vi "niFpga wdp fft DIF 4spc.vi"(0 "real data in":fxp<+/-,8,1>[](array[numeric])=[0.0, 0.0, 0.0, 0.0], 5 "imaginary data in":fxp<+/-,8,1>[](array[numeric])=[0.0, 0.0, 0.0, 0.0], 9 "input frame start":bool, 12 "enable":bool) -> (3 "data indices":u16[](array[numeric]), 4 "real data out":fxp<+,8,1>[](array[numeric]) format="%#.6g", 6 "imaginary data out":fxp<+,8,1>[](array[numeric]) format="%#.6g", 10 "output valid":bool, 14 "ready for frame":bool, 15 "output frame start":bool)   [LabVIEW 2017]
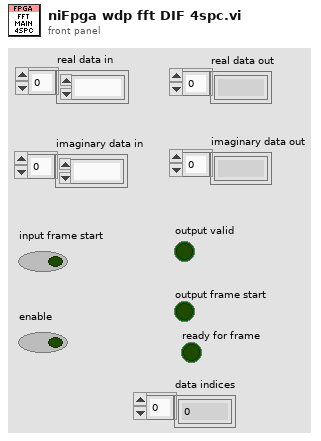
[diagram p1: front panel]
types:
  T1 = cluster{"internal input type":fxp<+/-,8,1>, "internal input type":fxp<+/-,8,1>}
  T2 = cluster{"internal input type":fxp<+/-,8,1>, "internal input type":fxp<+/-,8,1>}[]
  T3 = cluster{"x-y":fxp<+/-,20,13>, "x-y":fxp<+/-,20,13>}[]
  T4 = cluster{"data re":fxp<+/-,8,1>, "data im":fxp<+/-,8,1>}[]
  T5 = cluster{"data re":fxp<+/-,8,1>, "data im":fxp<+/-,8,1>}
  T6 = cluster{"twiddle factor type":fxp<+/-,16,2>, "twiddle factor type":fxp<+/-,16,2>}[]
  T7 = cluster{"x-y":fxp<+/-,19,12>, "x-y":fxp<+/-,19,12>}
  T8 = cluster{"x+y":fxp<+/-,19,12>, "x+y":fxp<+/-,19,12>}
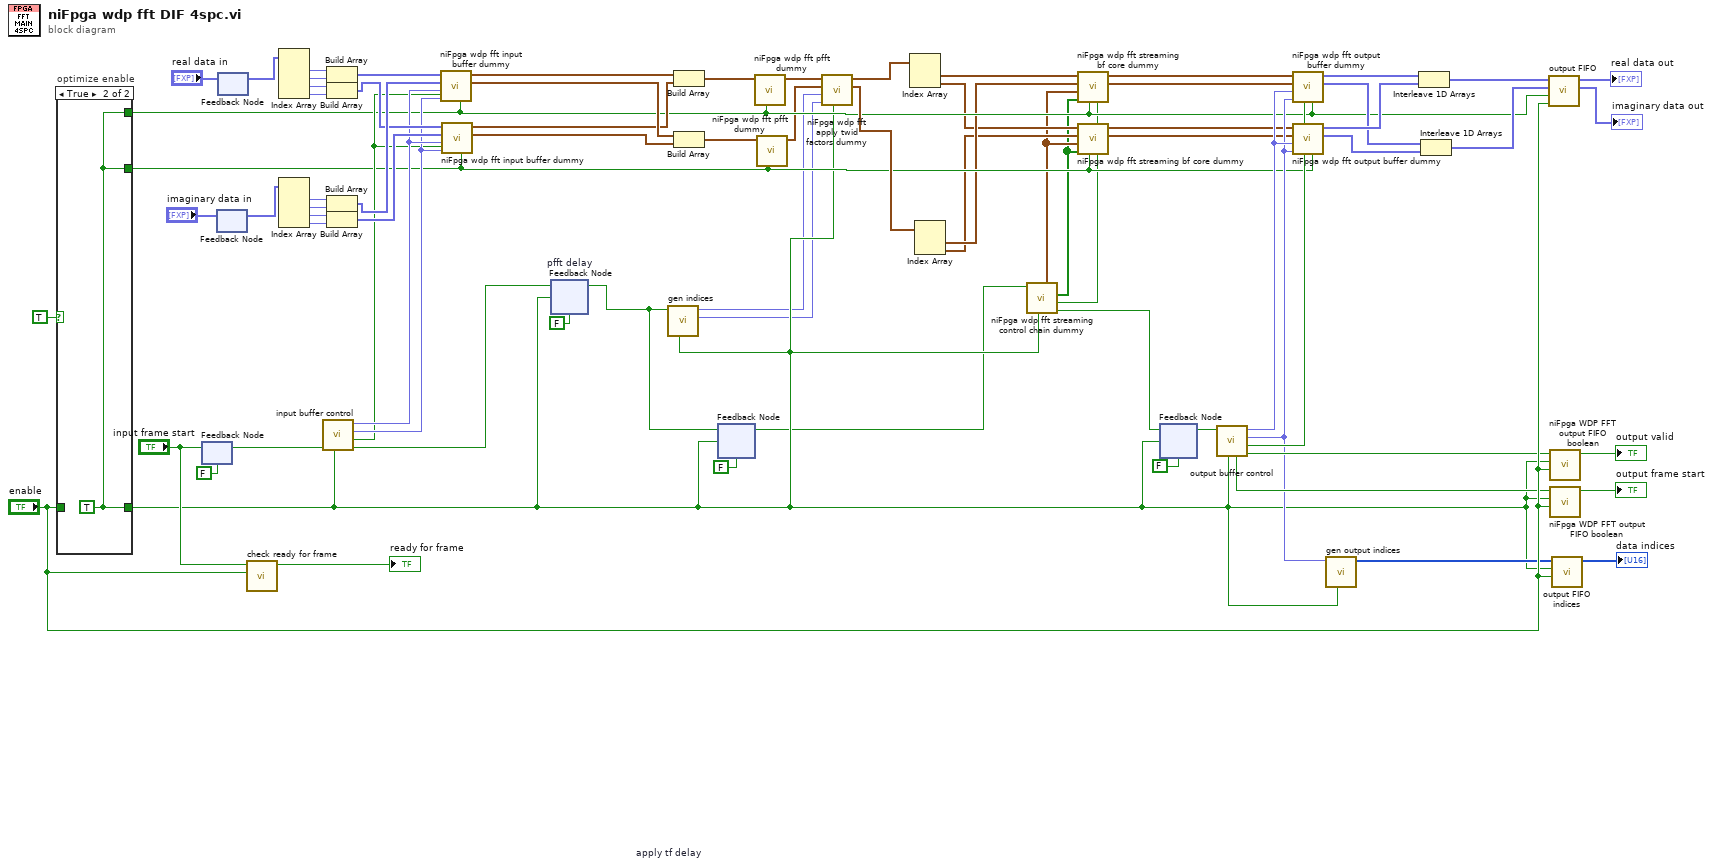
[diagram p0: block diagram]
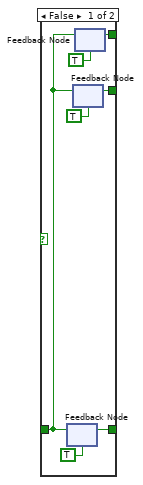
[diagram p2: hidden frame]
diagram:
  n1 = case "optimize enable" shown="True" TRUE {
    tunnel: [w81 w84] -> w18
    tunnel: "enable" -> [w79 _]
    tunnel: [w78 w84] -> w30
    tunnel: [w77 w84] -> w29
    frame False {
      n2 = feedback #1(TRUE ("enable")) -> (w81:bool)
      n3 = feedback-in #1(w79) -> ()
      n4 = feedback #2(TRUE ("enable")) -> (w77:bool)
      n5 = feedback-in #2(w79) -> ()
      n6 = feedback #3(TRUE ("enable")) -> (w78:bool)
      n7 = feedback-in #3(w79) -> ()
    }
    frame True {
      w84 = TRUE
    }
  }
  n8 = feedback #4(FALSE ("enable")) -> (w69:bool)
  n9 = feedback-in #4("input frame start") -> ()
  n10 = feedback #5() -> (w59:fxp<+/-,8,1>[])  [unwired: 1 in]
  n11 = feedback-in #5("imaginary data in") -> ()
  n12 = feedback #6() -> (w60:fxp<+/-,8,1>[])  [unwired: 1 in]
  n13 = feedback-in #6("real data in") -> ()
  n14 = call "check ready for frame"("enable"="enable", "frame start in"="input frame start") -> ("ready for frame"=→"ready for frame":bool)  [unwired: 9 in]
  n15 = Index Array(array=w60) -> (element #1=w14:fxp<+/-,8,1>, element #2=w13:fxp<+/-,8,1>, element #3=w12:fxp<+/-,8,1>, element #4=w11:fxp<+/-,8,1>)  [unwired: 4 in]
  n16 = Index Array(array=w59) -> (element #1=w7:fxp<+/-,8,1>, element #2=w8:fxp<+/-,8,1>, element #3=w9:fxp<+/-,8,1>, element #4=w10:fxp<+/-,8,1>)  [unwired: 4 in]
  n17 = call "input buffer control"("enable"=w18, "frame start in"=w69) -> ("frame start out"=w68:bool, "write memory 2?"=w43:bool, "read index"=w53:fxp<+,9,9>, "write index"=w54:fxp<+,8,8>)  [unwired: 6 in]
  n18 = Build Array(w14, w13) -> (w58:fxp<+/-,8,1>[])
  n19 = Build Array(w12, w11) -> (w56:fxp<+/-,8,1>[])
  n20 = Build Array(w7, w8) -> (w57:fxp<+/-,8,1>[])
  n21 = Build Array(w9, w10) -> (w55:fxp<+/-,8,1>[])
  n22 = call <vilib>:"niFpga wdp fft input buffer dummy.vi"("enable"=w30, "write memory 2?"=w43, "read index"=w53, "write index"=w54, "data in im"=w57, "data in re"=w58) -> ("data out 1"=w51:T1, "data out 0"=w52:T1)  [unwired: 4 in]
  n23 = call <vilib>:"niFpga wdp fft input buffer dummy.vi"("enable"=w29, "write memory 2?"=w43, "read index"=w53, "write index"=w54, "data in im"=w55, "data in re"=w56) -> ("data out 1"=w49:T1, "data out 0"=w50:T1)  [unwired: 4 in]
  n24 = feedback #7 "pfft delay"(FALSE) -> (w31:bool)
  n25 = feedback-in #7(w68, w18) -> ()
  n26 = call "gen indices"("enable"=w18, "frame start"=w31) -> ("data index 1"=w16:fxp<+,10,10>, "data index 0"=w17:fxp<+,10,10>)  [unwired: 8 in]
  n27 = Build Array(w52, w50) -> (w66:T2)
  n28 = Build Array(w51, w49) -> (w65:T2)
  n29 = feedback #8 "apply tf delay"(FALSE) -> (w15:bool)
  n30 = feedback-in #8(w31, w18) -> ()
  n31 = call <vilib>:"niFpga wdp fft pfft dummy.vi"("enable"=w30, "data in"=w66) -> ("data out"=w5:T3)  [unwired: 9 in]
  n32 = call <vilib>:"niFpga wdp fft pfft dummy.vi"("enable"=w29, "data in"=w65) -> ("data out"=w4:T3)  [unwired: 9 in]
  n33 = call <vilib>:"niFpga wdp fft apply twid factors dummy.vi"("enable"=w18, "data index 1"=w16, "data index 0"=w17, "data in 1"=w4, "data in 0"=w5) -> ("data out 1"=w75:T4, "data out 0"=w76:T4)  [unwired: 5 in]
  n34 = Index Array(array=w76) -> (element #1=w28:T5, element #2=w24:T5)  [unwired: 2 in]
  n35 = Index Array(array=w75) -> (element #1=w26:T5, element #2=w22:T5)  [unwired: 2 in]
  n36 = call <vilib>:"niFpga wdp fft streaming control chain dummy.vi"("enable"=w18, "input frame start"=w15) -> ("frame start"=w20:bool, "index=0?"=w1:bool, "switch"=w2:bool[], "twiddle factors"=w3:T6)  [unwired: 5 in, 1 out]
  n37 = call <vilib>:"niFpga wdp fft streaming bf core dummy.vi"("index=0?"=w1, "enable"=w30, "switch"=w2, "twiddle factors"=w3, "data in 1"=w26, "data in 0"=w28) -> ("data out 1"=w25:T7, "data out 0"=w27:T8)  [unwired: 4 in]
  n38 = call <vilib>:"niFpga wdp fft streaming bf core dummy.vi"("index=0?"=w1, "enable"=w29, "switch"=w2, "twiddle factors"=w3, "data in 1"=w22, "data in 0"=w24) -> ("data out 1"=w21:T7, "data out 0"=w23:T8)  [unwired: 4 in]
  n39 = feedback #9 ("delay")(FALSE) -> (w19:bool)
  n40 = feedback-in #9(w20, w18) -> ()
  n41 = call "output buffer control"("enable"=w18, "frame start"=w19) -> ("output valid?"=w38:bool, "memory switch"=w36:bool, "read index"=w35:fxp<+,4,4>, "write index"=w37:fxp<+,9,9>, "frame start?"=w39:bool)  [unwired: 5 in]
  n42 = call <vilib>:"niFpga wdp fft output buffer dummy.vi"("enable"=w30, "memory switch"=w36, "read index"=w35, "write index"=w37, "data in 1"=w25, "data in 0"=w27) -> ("data out im"=w62:fxp<+/-,32,16>[], "data out re"=w64:fxp<+/-,32,16>[])  [unwired: 4 in]
  n43 = call <vilib>:"niFpga wdp fft output buffer dummy.vi"("enable"=w29, "memory switch"=w36, "read index"=w35, "write index"=w37, "data in 1"=w21, "data in 0"=w23) -> ("data out im"=w61:fxp<+/-,32,16>[], "data out re"=w63:fxp<+/-,32,16>[])  [unwired: 4 in]
  n44 = call "gen output indices"("enable"=w18, "index"=w35) -> ("data indices"=w34:u16[])  [unwired: 9 in]
  n45 = Interleave 1D Arrays(w64, w63) -> (w47:fxp<+/-,32,16>[])
  n46 = Interleave 1D Arrays(w62, w61) -> (w46:fxp<+/-,32,16>[])
  n47 = call "output FIFO"("enable"="enable", "enable with delay"=w30, "data in 1"=w46, "data in 0"=w47) -> ("data out 1"=→"imaginary data out":fxp<+,8,1>[], "data out 0"=→"real data out":fxp<+,8,1>[])  [unwired: 6 in]
  n48 = call <vilib>:"niFpga WDP FFT output FIFO boolean.vi"("enable"="enable", "enable with delay"=w18, "boolean in"=w38) -> ("boolean out"=→"output valid":bool)  [unwired: 8 in]
  n49 = call <vilib>:"niFpga WDP FFT output FIFO boolean.vi"("enable"="enable", "enable with delay"=w18, "boolean in"=w39) -> ("boolean out"=→"output frame start":bool)  [unwired: 8 in]
  n50 = call "output FIFO indices"("enable"="enable", "enable with delay"=w18, "data in"=w34) -> ("data out"=→"data indices":u16[])  [unwired: 8 in]
